vi "UpdateParentMap.vi"(8 "error in (no error)":errorcluster, 11 "MailboxManager in":refnum<class "MailboxManager.lvclass">) -> (0 "error out":errorcluster, 3 "MailboxManager out":refnum<class "MailboxManager.lvclass">)   [LabVIEW 2020, in "MailboxManager.lvlib" / "MailboxManager.lvclass"]
uses:
  MailboxManager.lvclass
  MailboxManager.lvclass/MailboxManager.ctl
  <vilib>/ActorFramework/Message Enqueuer/Message Enqueuer.lvclass
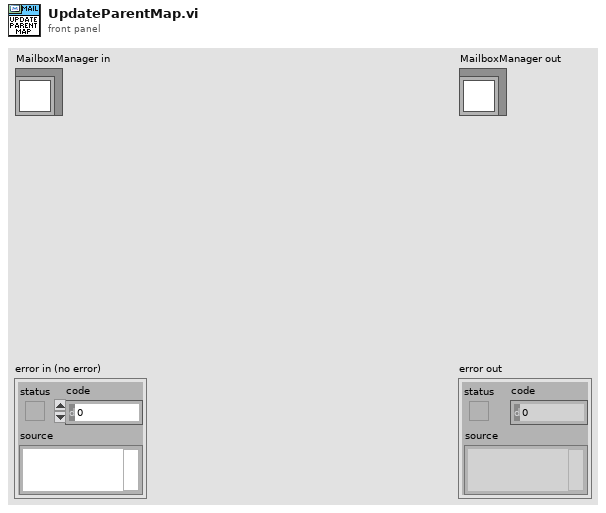
[diagram p1: front panel]
types:
  T1 = map{refnum<class "MailBoxMessage.lvclass">, refnum<class "Message Enqueuer.lvclass">[]}
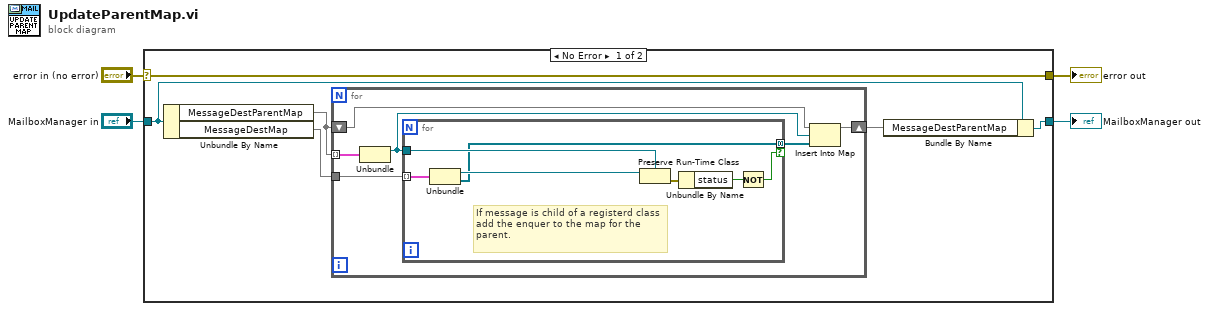
[diagram p0: block diagram]
diagram:
  n1 = case shown="No Error" "error in (no error)" {
    selector: "error in (no error)" -> [w10 w25]
    tunnel: [w10 w25] -> w3
    tunnel: [w6 w24] -> w1
    tunnel: "MailboxManager in" -> [w9 w24]
    frame No Error {
      n2 = Unbundle By Name(w9) -> ("MessageDestParentMap"=w7:T1, "MessageDestMap"=w8:T1)
      n3 = for {
        tunnel: w7 -> [w16] mode=indexing
        tunnel: w8 -> [w15]
        shift-right: [w14] -> w5
        shift-left: w7 -> [w12]
        n4 = Unbundle(w16) -> ("MailBoxMessage"=w13:refnum<class "MailBoxMessage.lvclass">)  [unwired: 1 out]
        n5 = for {
          tunnel: w13 -> [w21]
          tunnel: w15 -> [w20] mode=indexing
          tunnel: [w18] -> w11 mode=concatenating if=w17
          # "If message is child of a registerd class add the enquer to the map for the parent."
          n6 = Unbundle(w20) -> ("MailBoxMessage"=w19:refnum<class "MailBoxMessage.lvclass">, "Message Enqueuers"=w18:refnum<class "Message Enqueuer.lvclass">[])
          n7 = Preserve Run-Time Class(object in=w19, 2:w21) -> (error out=w22:errorcluster)  [unwired: 1 in, 1 out]
          n8 = Unbundle By Name(w22) -> ("status"=w23:bool)
          n9 = Not(x=w23) -> (.not. x?=w17:bool)
        }
        n10 = Insert Into Map(map in=w12, key=w13, value=w11) -> (map out=w14:T1)  [unwired: 2 out]
      }
      n11 = Bundle By Name(cluster=w9, "MessageDestParentMap"=w5) -> (w6:refnum<class "MailboxManager.lvclass">)
    }
    frame Error {
    }
  }
  "error out" <- w3
  "MailboxManager out" <- w1
